vi "Uniform CDF.vi"(9 "xmax":dbl=1.0, 10 "xmin":dbl, 11 "x":dbl) -> (0 "error":i32, 3 "cdf(x)":dbl=1.0)   [LabVIEW 2010, in "NI_Gmath.lvlib"]
doc: "Computes the continuous cumulative distribution function (CDF), or the probability that the random variate X, where X describes the selected distribution type, has a value less than or equal to <B>x</B>. You must manually select the polymorphic instance to use."
uses:
  NI_Gmath.lvlib
  st_error_code.ctl
panel:
  # "Uniform CDF"
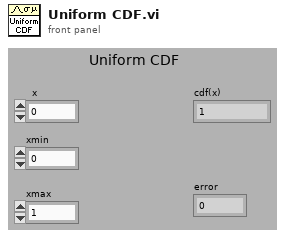
[diagram p1: front panel]
types:
  T1 = typedef "NI_Gmath.lvlib/st_error_code.ctl" = i32
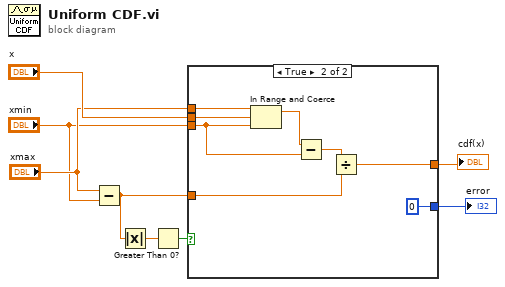
[diagram p0: block diagram]
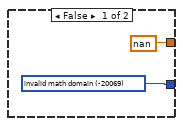
[diagram p2: hidden frame]
diagram:
  n1 = Subtract(x="xmax", y="xmin") -> (x-y=w4:dbl)
  n2 = Absolute Value(x=w4) -> (abs(x)=w5:dbl)
  n3 = Greater Than 0?(x=w5) -> (x > 0?=w3:bool)
  n4 = case shown="True" w3 {
    tunnel: "x" -> [_ w17]
    tunnel: "xmax" -> [_ w16]
    tunnel: "xmin" -> [_ w15]
    tunnel: w4 -> [_ w12]
    tunnel: [nan w13] -> w2
    tunnel: [w9 0] -> w1
    frame False {
      w9 = T1 -20069 items=["invalid math domain"=-20069, "Fourier interpolation size m >= n"=-20070, "empty array"=-20003] ("stat interp error code")
    }
    frame True {
      n5 = In Range and Coerce(upper limit=w16, x=w17, lower limit=w15) -> (coerced(x)=w11:dbl)  [unwired: 1 out]
      n6 = Subtract(x=w11, y=w15) -> (x-y=w14:dbl)
      n7 = Divide(x=w14, y=w12) -> (x/y=w13:dbl)
    }
  }
  "cdf(x)" <- w2
  "error" <- w1
